vi "Find Properties that apply to Object.vi"(11 "GObject in":refnum<vi>) -> (3 "Relevant Properties":string[](array[string]))   [LabVIEW 2019, in "LSS.lvlib"]
doc: "Generate a list of properties that apply to the control reference input. This is used while setting up style sheets as an aide to know which properties apply. This VI must be updated manually for any new properties that are added to LSS.\n\n<b>Inputs:</b>\n<b>GObject in</b> - Object to find the applicable styles list for.\n\n<b>Outputs:</b> \n<b>Relevent Properties</b> - List of properties that apply to the control input."
uses:
  LSS.lvlib
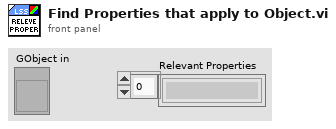
[diagram p1: front panel]
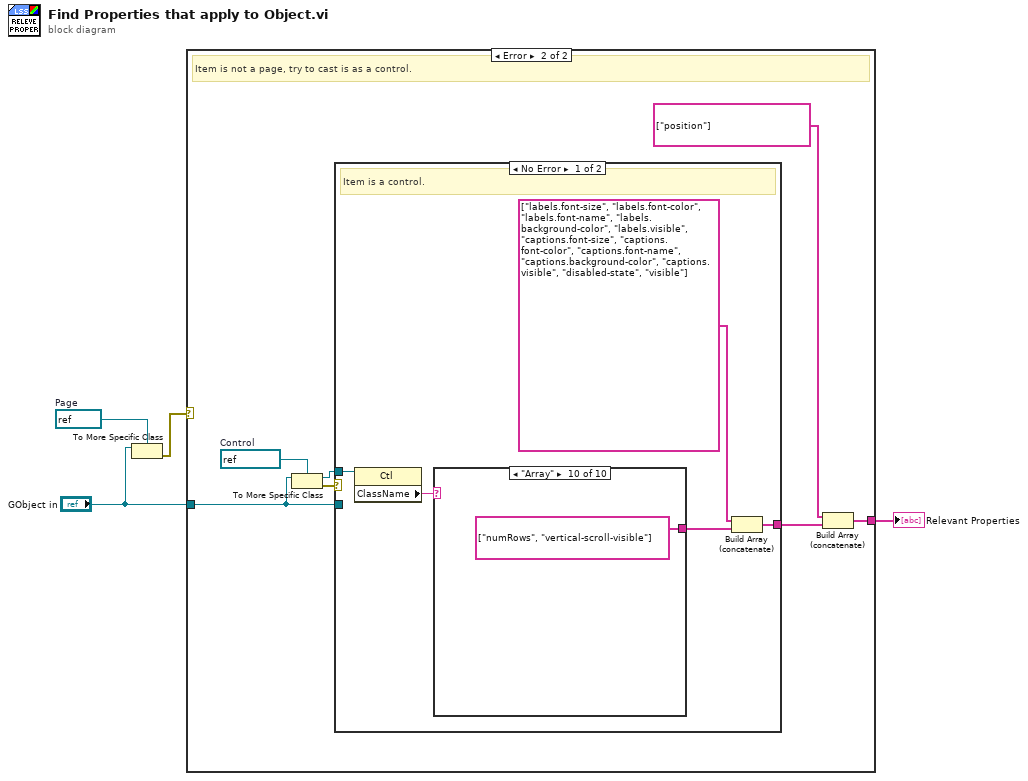
[diagram p0: block diagram]
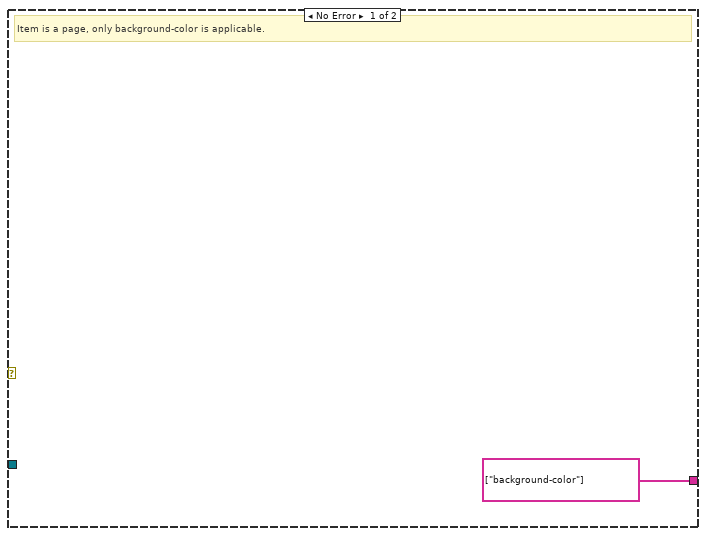
[diagram p2: hidden frame]
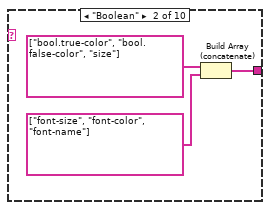
[diagram p4: hidden frame]
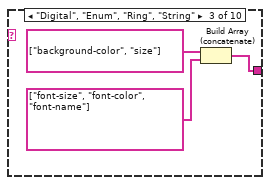
[diagram p5: hidden frame]
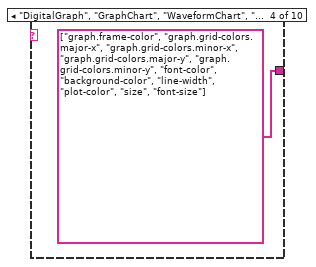
[diagram p6: hidden frame]
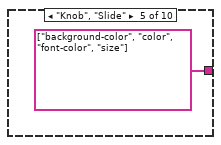
[diagram p7: hidden frame]
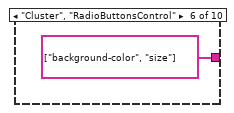
[diagram p8: hidden frame]
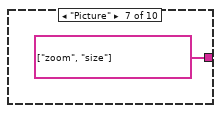
[diagram p9: hidden frame]
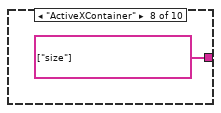
[diagram p10: hidden frame]
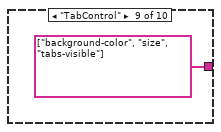
[diagram p11: hidden frame]
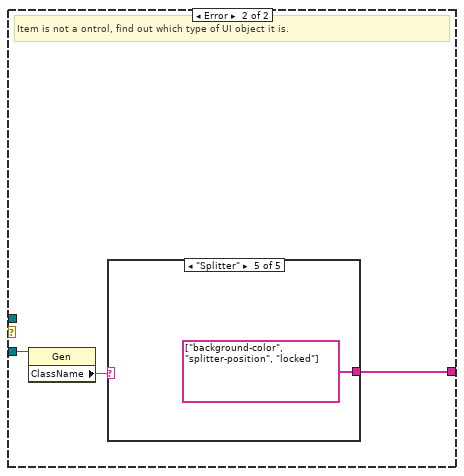
[diagram p12: hidden frame]
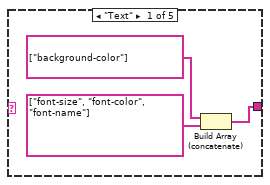
[diagram p13: hidden frame]
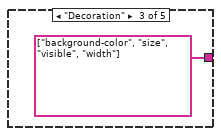
[diagram p15: hidden frame]
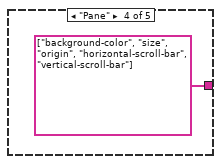
[diagram p16: hidden frame]
diagram:
  w2 = refnum<vi> refnum  # Page
  n1 = To More Specific Class(target class=w2, reference="GObject in") -> (error out=w1:errorcluster)  [unwired: 1 in, 1 out]
  n2 = case shown="Error" w1 {
    tunnel: "GObject in" -> [_ w10]
    tunnel: [string[] ["background-color"] w6] -> w4
    frame No Error {
      # "Item is a page, only background-color is applicable."
    }
    frame Error {
      w12 = refnum<vi> refnum  # Control
      # "Item is not a page, try to cast is as a control."
      n3 = To More Specific Class(target class=w12, reference=w10) -> (specific class reference=w9:refnum<vi>, error out=w11:errorcluster)  [unwired: 1 in]
      n4 = case shown="No Error" w11 {
        tunnel: w10 -> [_ w33]
        tunnel: [w13 w31] -> w8
        tunnel: w9 -> [w17 _]
        frame No Error {
          # "Item is a control."
          n5 = property class="Ctl"(reference=w17) -> ("ClassName"=w16:string)  [unwired: 1 in, 2 out]
          n6 = case shown="\"Array\"" w16 {
            tunnel: [_ w20 w23 string[] ["graph.frame-color", "graph.grid-colors.major-x", "graph.grid-colors.minor-x", "graph.grid-colors.major-y", "graph.grid-colors.minor-y", "font-color", "background-color", "line-width", "plot-color", "size", "font-size"] string[] ["background-color", "color", "font-color", "size"] string[] ["background-color", "size"] string[] ["zoom", "size"] string[] ["size"] string[] ["background-color", "size", "tabs-visible"] string[] ["numRows", "vertical-scroll-visible"]] -> w14
            frame Default {
            }
            frame "Boolean" {
              n7 = Build Array (concatenate)(string[] ["bool.true-color", "bool.false-color", "size"], string[] ["font-size", "font-color", "font-name"]) -> (w20:string[])
            }
            frame "Digital", "Enum", "Ring", "String" {
              n8 = Build Array (concatenate)(string[] ["background-color", "size"], string[] ["font-size", "font-color", "font-name"]) -> (w23:string[])
            }
            frame "DigitalGraph", "GraphChart", "WaveformChart", "WaveformGraph", "XYGraph" {
            }
            frame "Knob", "Slide" {
            }
            frame "Cluster", "RadioButtonsControl" {
            }
            frame "Picture" {
            }
            frame "ActiveXContainer" {
            }
            frame "TabControl" {
            }
            frame "Array" {
            }
          }
          n9 = Build Array (concatenate)(string[] ["labels.font-size", "labels.font-color", "labels.font-name", "labels.background-color", "labels.visible", "captions.font-size", "captions.font-color", "captions.font-name", "captions.background-color", "captions.visible", "disabled-state", "visible"], w14) -> (w13:string[])
        }
        frame Error {
          # "Item is not a ontrol, find out which type of UI object it is."
          n10 = property class="Gen"(reference=w33) -> ("ClassName"=w32:string)  [unwired: 1 in, 2 out]
          n11 = case shown="\"Splitter\"" w32 {
            tunnel: [w34 _ string[] ["background-color", "size", "visible", "width"] string[] ["background-color", "size", "origin", "horizontal-scroll-bar", "vertical-scroll-bar"] string[] ["background-color", "splitter-position", "locked"]] -> w31
            frame "Text" {
              n12 = Build Array (concatenate)(string[] ["background-color"], string[] ["font-size", "font-color", "font-name"]) -> (w34:string[])
            }
            frame Default {
            }
            frame "Decoration" {
            }
            frame "Pane" {
            }
            frame "Splitter" {
            }
          }
        }
      }
      n13 = Build Array (concatenate)(string[] ["position"], w8) -> (w6:string[])
    }
  }
  "Relevant Properties" <- w4
